vi "ScanString.vi"(8 "error in (no error)":errorcluster, 10 "String":string, 11 "Float D Element in":refnum<class "Float D Element.lvclass">) -> (0 "error out":errorcluster, 3 "Float D Element out":refnum<class "Float D Element.lvclass">)   [LabVIEW 2020, in "D Datagrid Library.lvlib" / "Float D Element.lvclass"]
uses:
  Float D Element.lvclass
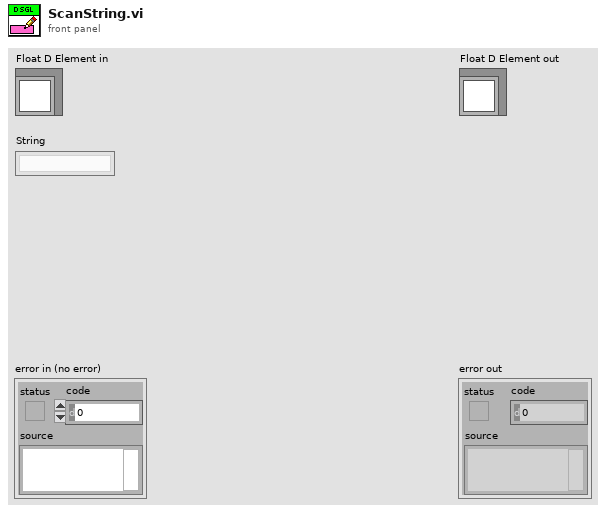
[diagram p1: front panel]
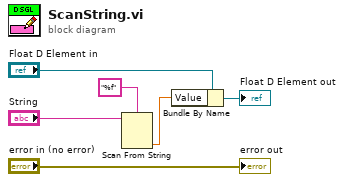
[diagram p0: block diagram]
diagram:
  n1 = Scan From String(format string="%f", input string="String") -> (output 1=w2:dbl)  [unwired: 3 in, 3 out]
  n2 = Bundle By Name(cluster="Float D Element in", "Value"=w2) -> (→"Float D Element out":refnum<class "Float D Element.lvclass">)
  "error out" <- "error in (no error)"
